vi "3D-DrawPictureB.vi"(8 "error in (no error)":errorcluster, 9 "Labstringarray":string[](array[string]), 10 "ROI Array":T1[](array[typedef]) {"Rotation" format="%.2f"; "Left" scale=0.0..1024.0; "Right" scale=0.0..1024.0}, 11 "A Demo in":T2(plugin-control)) -> (0 "error out":errorcluster, 3 "A Demo out":T2(plugin-control))   [LabVIEW 2015]
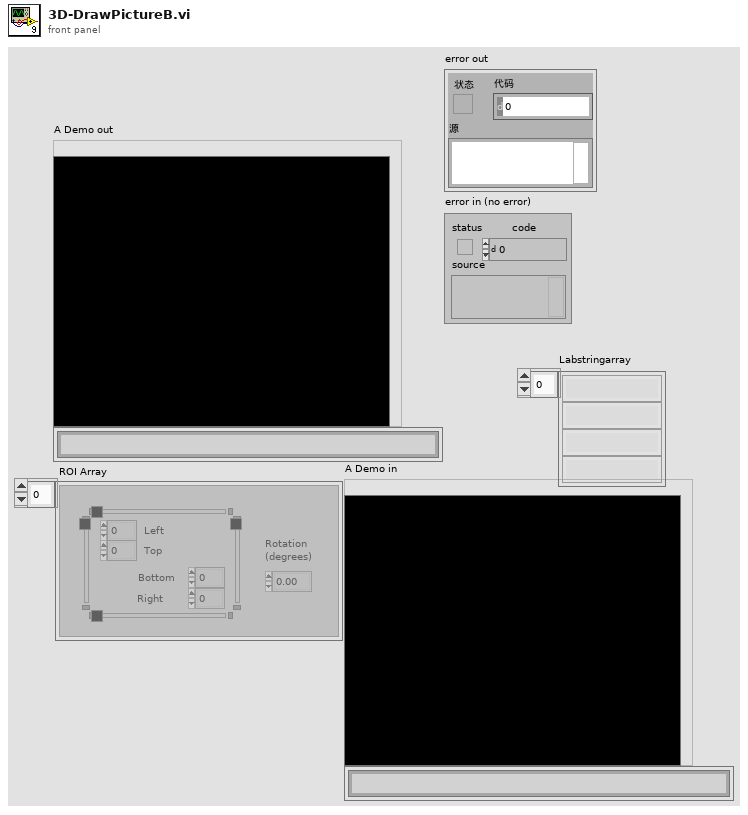
[diagram p1: front panel]
types:
  T1 = typedef "IMAQ Rectangle" = cluster{"Left":i32, "Top":i32, "Right":i32, "Bottom":i32, "Rotation":dbl}
  T2 = typedef "IMAQ Image.ctl" = refnum<image>
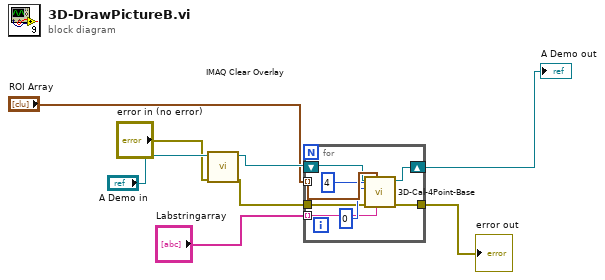
[diagram p0: block diagram]
diagram:
  n1 = call "IMAQ Clear Overlay"("error in (no error)"="error in (no error)", "Image"="A Demo in") -> ("error out"=w6:errorcluster, "Image Out"=w7:T2)  [unwired: 8 in]
  n2 = for {
    tunnel: "ROI Array" -> [w16] mode=indexing
    tunnel: w6 -> [w11]
    tunnel: [w10] -> w5
    tunnel: "Labstringarray" -> [w9] mode=indexing
    shift-right: [w14] -> w4
    shift-left: w7 -> [w15]
    n3 = call "3D-Cal-4Point-Base.vi"("Labstring"=w9, "Rectangle"=w16, "error in (no error)"=w11, "十字线距离"=4, "基准点距离"=0, "Pic Input"=w15) -> ("error out"=w10:errorcluster, "Pic Output"=w14:T2)  [unwired: 3 in, 1 out]
  }
  "A Demo out" <- w4
  "error out" <- w5
